vi "Configure RemIO Module Core.vi"(8 "error in (no error)":errorcluster, 9 "module slot index":u8=1, 10 "Slave Ref In":refnum<k21>, 11 "11100 in":refnum<class "11100.lvclass">) -> (0 "error out":errorcluster, 1 "negative confirmation":T1 {"additional error code" format="%.0x"; "error code" format="%.0x"}, 2 "Slave Ref Out":refnum<k21>, 3 "11100 out":refnum<class "11100.lvclass">, 5 "SDO abort code":u32 format="%.0x")   [LabVIEW 2020, in "Modules.lvlib" / "11100.lvclass"]
uses:
  11100.lvclass
  <vilib>/indcomecat/Remote IO/typedefs/negative confirmation.ctl
  11100.lvclass/11100.ctl
  c288c884-db83-4801-86c2-0691c86b7e02.vi
  RemIO Module/Get RemIO Library Path.vi
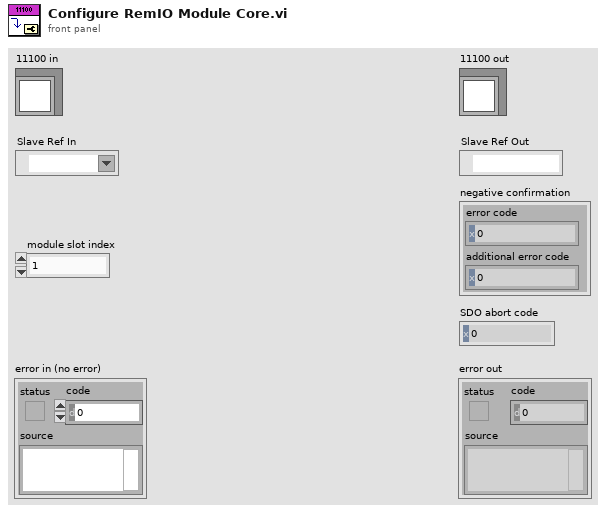
[diagram p1: front panel]
types:
  T1 = typedef "negative confirmation.ctl" = cluster{"error code":u16, "additional error code":u16}
  T2 = typedef "NI ECAT Remote IO.lvlib/channel number REM-11100.ctl" = u8
  T3 = typedef "NI ECAT Remote IO.lvlib/input filter time REM-11100.ctl" = u8
  T4 = typedef "NI ECAT Remote IO.lvlib/mean-value REM-11100.ctl" = u8
  T5 = typedef "NI ECAT Remote IO.lvlib/measuring range REM-11100.ctl" = u8
  T6 = cluster{"channel number":T2, "input filter time":T3, "mean-value":T4, "measuring range":T5}[]
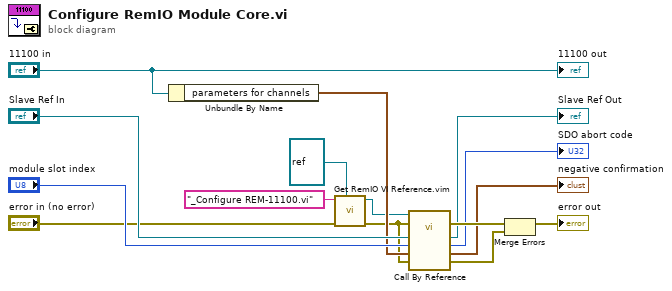
[diagram p0: block diagram]
diagram:
  n1 = Unbundle By Name("11100 in") -> ("parameters for channels"=w12:T6)
  n2 = call "Get RemIO VI Reference.vim"("name or relative path"="_Configure REM-11100.vi", "error in (no error)"="error in (no error)", "type specifier VI Refnum (for type only)"=refnum<vi> refnum) -> ("vi reference"=w3:refnum<vi>, "error out"=w4:errorcluster)  [unwired: 6 in]
  n3 = call-by-ref "?"(reference=w3, error in=w4, 8:"error in (no error)"=w4, "parameters for channels"=w12, "module slot index"="module slot index", "slave reference in"="Slave Ref In") -> (error out=w10:errorcluster, 0:"error out"=w11:errorcluster, "negative confirmation"=→"negative confirmation":T1, "SDO abort code"=→"SDO abort code":u32, "slave reference out"=→"Slave Ref Out":refnum<k21>)  [unwired: 4 in, 1 out]
  n4 = Merge Errors(w10, w11) -> (→"error out":errorcluster)
  "11100 out" <- "11100 in"
